vi "Fire_Sequence_State_Machine_12_13.vi"(1 "PT Filepath":path=path "D:/PDE Project/PDE Data/Default Data/PT.tdms", 2 "TC Filepath":path=path "D:/PDE Project/PDE Data/Default Data/TC.tdms", 3 "PD Filepath":path=path "test.tdms" caption="Filename", 8 "Data Time":dbl=1.0 min=0.0 max=120.0, 9 "Purge":bool, 10 "Save Data":bool, 11 "Stop Button":bool) -> (0 "Enum":T1=enum."PDE Inject", 4 "Error Out":errorcluster)   [LabVIEW 2017]
uses:
  FireProc.ctl
  <vilib>/DAQmx/read.llb/DAQmx Read (Analog 1D Wfm NChan NSamp).vi
  <vilib>/DAQmx/create/channels.llb/DAQmx Create Channel (AI-Voltage-Basic).vi
  <vilib>/DAQmx/configure/timing.llb/DAQmx Timing (Sample Clock).vi
  <vilib>/DAQmx/configure/trigger.llb/DAQmx Start Trigger (Digital Edge).vi
  <vilib>/DAQmx/configure/trigger.llb/DAQmx Reference Trigger (Digital Edge).vi
  <vilib>/DAQmx/miscellaneous.llb/DAQmx Fill In Error Info.vi
  <resource>/objmgr/daqmx.rc
panel:
  out "Saving Data":bool
  in  "error in":errorcluster
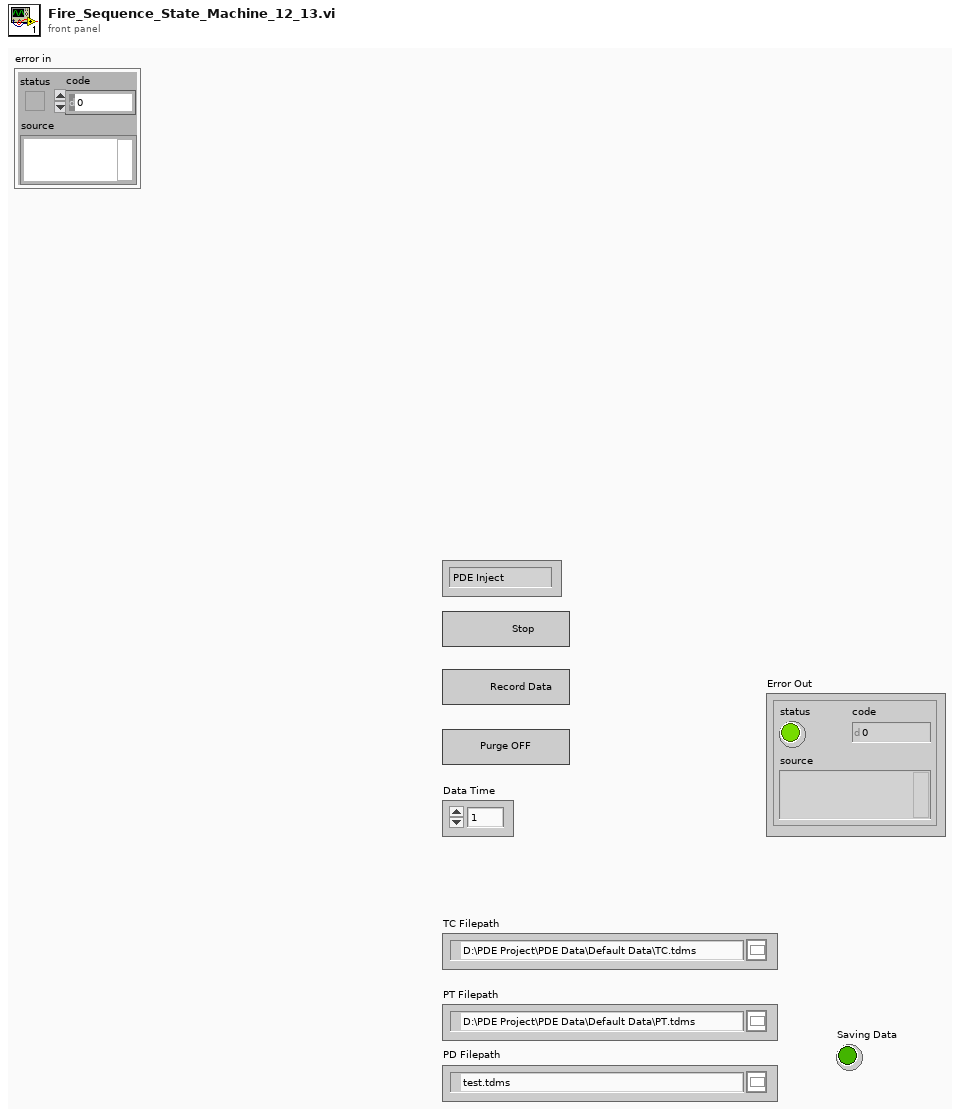
[diagram p1: front panel]
types:
  T1 = typedef "FireProc.ctl" = enum16{"Purge", "Ignite", "Predet Inject", "PDE Inject", "Stop"}
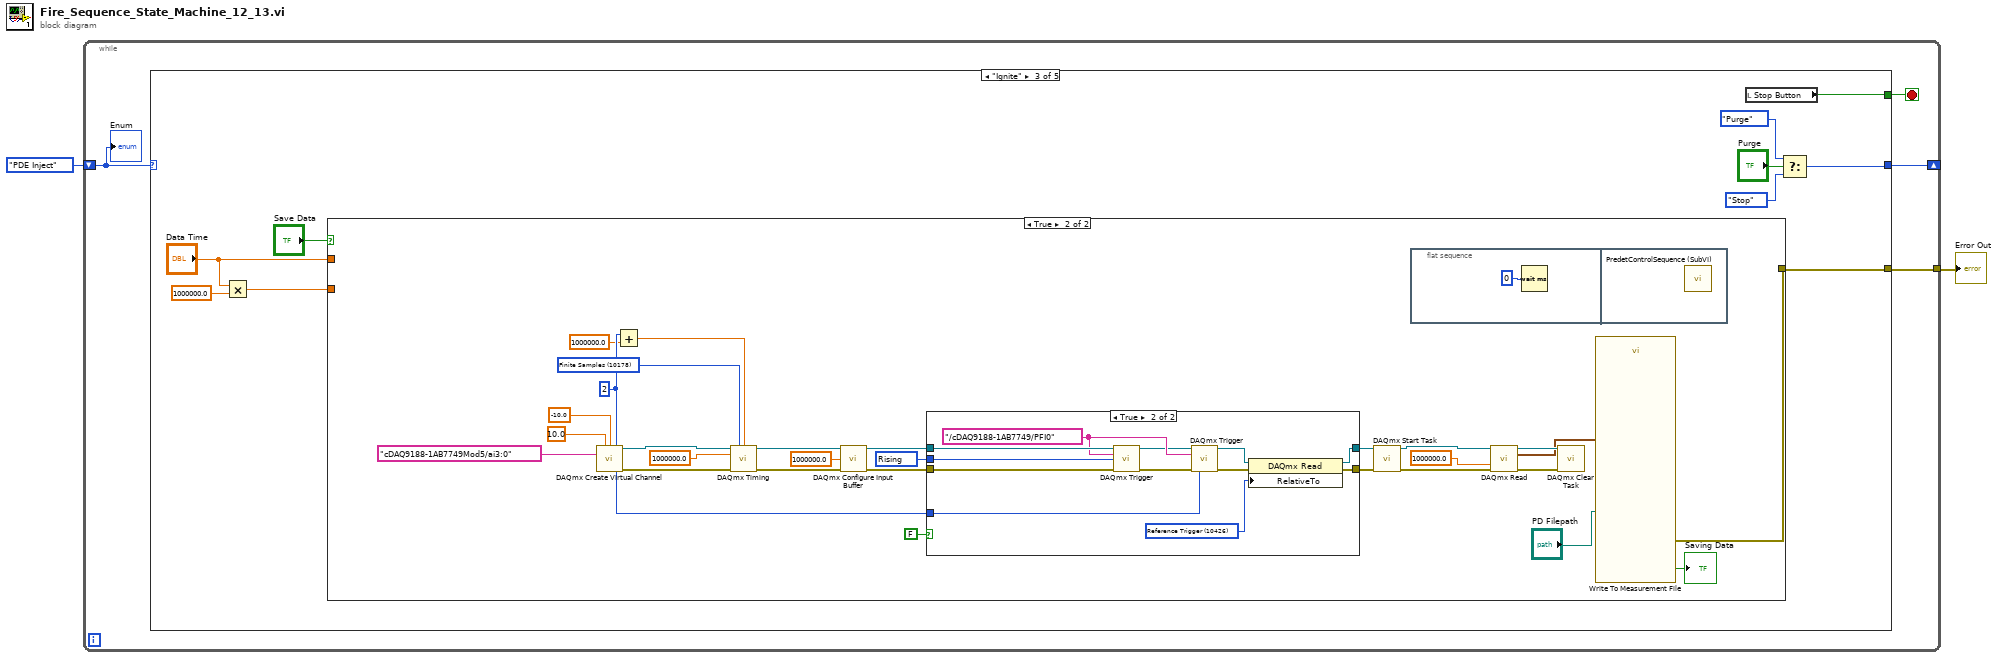
[diagram p0: block diagram]
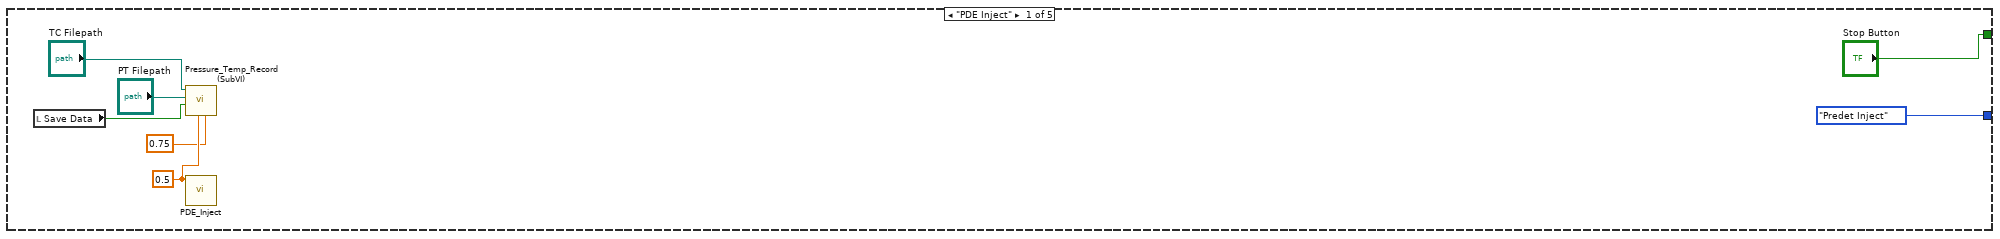
[diagram p2: hidden frame]
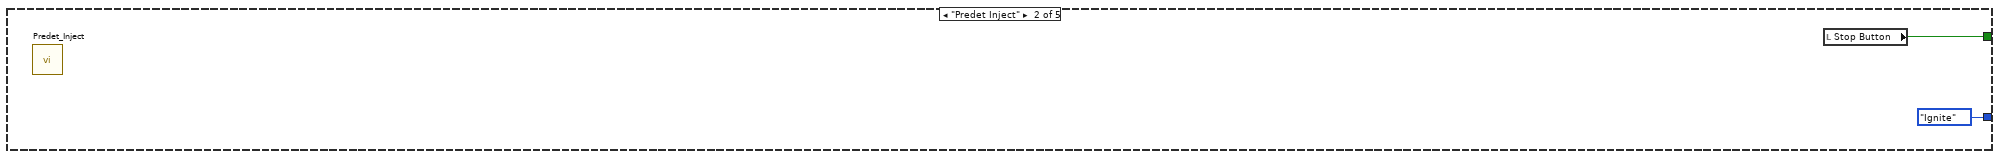
[diagram p3: hidden frame]
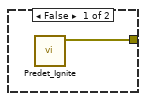
[diagram p4: hidden frame]
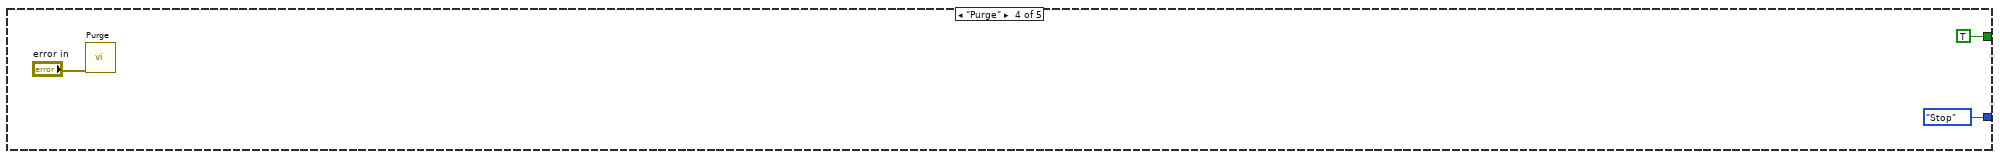
[diagram p6: hidden frame]
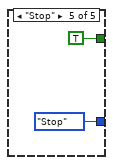
[diagram p7: hidden frame]
diagram:
  n1 = while {
    shift-right: [w6] -> _
    shift-left: FireProc."PDE Inject" -> [w4]
    tunnel: [w3] -> w1
    stop <- w5 stop-if-true
    n2 = case shown="\"Ignite\"" w4 {
      tunnel: [FireProc."Predet Inject" FireProc."Ignite" w22 FireProc."Stop" FireProc."Stop"] -> w6
      tunnel: ["Stop Button" w14 w20 TRUE TRUE ("Stop Button")] -> w5
      tunnel: [_ _ w16 _ _] -> w3
      frame "PDE Inject" {
        w11 = 0.5 ("Rate")
        n3 = local read "Save Data"() -> (w7:bool)
        n4 = call "Pressure_Temp_Record (SubVI).vi"("Delay Time (s)"=0.75, "Rate"=w11, "Save Data"=w7, "PT Filepath"="PT Filepath", "TC Filepath"="TC Filepath") -> ()  [unwired: 7 in]
        n5 = call "PDE_Inject.vi"("Rate"=w11) -> ()  [unwired: 10 in, 1 out]
      }
      frame "Predet Inject" {
        n6 = call "Predet_Inject.vi"() -> ()  [unwired: 12 in]
        n7 = local read "Stop Button"() -> (w14:bool)
      }
      frame "Ignite" {
        n8 = Multiply(x="Data Time", y=1000000.0 ("rate")) -> (x*y=w24:dbl)
        n9 = case shown="True" "Save Data" {
          tunnel: w24 -> [_ _]
          tunnel: "Data Time" -> [_ _]
          tunnel: [w26 w27] -> w16
          frame False {
            n10 = call "Predet_Ignite.vi"() -> ("Error Out"=w26:errorcluster)  [unwired: 10 in, 1 out]
          }
          frame True {
            w35 = 10280 items=["Rising"=10280, "Falling"=10171] ("edge")
            w37 = 10178 items=["Finite Samples"=10178, "Continuous Samples"=10123, "Hardware Timed Single Point"=12522] ("sample mode")
            w40 = 2
            n11 = call-poly <vilib>:"DAQmx Create Virtual Channel.vi"("maximum value"=10.0, "minimum value"=-10.0, "physical channels"=tag "cDAQ9188-1AB7749Mod5/ai3:0") -> ("task out"=w47:refnum<k21>, "error out"=w52:errorcluster)  [unwired: 11 in]
            n12 = Add(x=w40, y=1000000.0) -> (x+y=w38:dbl)
            n13 = call-poly <vilib>:"DAQmx Timing.vi"("task/channels in"=w47, "sample mode"=w37, "samples per channel"=w38, "rate"=1000000.0, "error in"=w52) -> ("task out"=w48:refnum<k21>, "error out"=w51:errorcluster)  [unwired: 9 in]
            n14 = call <vilib>:"DAQmx Configure Input Buffer.vi"("task/channels in"=w48, "buffer size (in samples per channel)"=1000000.0, "error in"=w51) -> ("task out"=w49:refnum<k21>, "error out"=w50:errorcluster)  [unwired: 11 in]
            n15 = case shown="True" FALSE {
              tunnel: w50 -> [w56 w69]
              tunnel: w49 -> [w57 w68]
              tunnel: [w57 w67] -> w46
              tunnel: [w56 w66] -> w45
              tunnel: w40 -> [_ w62]
              tunnel: w35 -> [_ w61]
              frame False {
              }
              frame True {
                w60 = tag "/cDAQ9188-1AB7749/PFI0" ("source")
                w63 = 10426 items=["First Sample"=10424, "Current Read Position"=10425, "Reference Trigger"=10426, "First Pretrigger Sample"=10427, "Most Recent Sample"=10428] ("RelativeTo")
                n16 = call-poly <vilib>:"DAQmx Trigger.vi"("task/channels in"=w68, "source"=w60, "edge"=w61, "error in"=w69) -> ("task out"=w59:refnum<k21>, "error out"=w58:errorcluster)  [unwired: 10 in]
                n17 = call-poly <vilib>:"DAQmx Trigger.vi"("task/channels in"=w59, "source"=w60, "error in"=w58, "pretrigger samples per channel"=w62) -> ("task out"=w65:refnum<k21>, "error out"=w64:errorcluster)  [unwired: 10 in]
                n18 = property class="DAQmx Read"(reference=w65, error in=w64, "RelativeTo"=w63) -> (reference out=w67:refnum<k21>, error out=w66:errorcluster)
              }
            }
            n19 = call <vilib>:"DAQmx Start Task.vi"("task/channels in"=w46, "error in"=w45) -> ("task out"=w32:refnum<k21>, "error out"=w33:errorcluster)  [unwired: 12 in]
            n20 = flat-sequence {
              frame #0 {
                n21 = Wait (ms)(milliseconds to wait=u32 0) -> ()  [unwired: 1 out]
              }
              frame #1 {
                n22 = call "PredetControlSequence (SubVI).vi"() -> ()  [unwired: 11 in, 1 out]
              }
            }
            n23 = call-poly <vilib>:"DAQmx Read.vi"("task/channels in"=w32, "timeout"=1000000.0, "error in"=w33) -> ("task out"=w30:refnum<k21>, "data"=w29:waveform(dbl)[], "error out"=w31:errorcluster)  [unwired: 10 in]
            n24 = call <vilib>:"DAQmx Clear Task.vi"("task in"=w30, "error in"=w31) -> ()  [unwired: 13 in, 1 out]
            n25 = call "Write To Measurement File"("Signals"=w29, "Filename"="PD Filepath") -> ("Saving Data"=→"Saving Data":bool, "error out"=w27:errorcluster)  [unwired: 15 in, 1 out]
          }
        }
        n26 = local read "Stop Button"() -> (w20:bool)
        n27 = Select(t=FireProc."Purge", s="Purge", f=FireProc."Stop") -> (s? t:f=w22:T1)
      }
      frame "Purge" {
        n28 = call "Purge.vi"("error in (no error)"="error in") -> ()  [unwired: 11 in]
      }
      frame "Stop" {
      }
    }
    "Enum" <- w4
  }
  "Error Out" <- w1
